vi "Set Current.vi"(4 "Factor (50.00) (EIN)":dbl=50.0, 6 "A Sensor Ratio(mV/A) (10.0000)":dbl=10.0 min=0.0001 max=99999.9999 step=0.0001 format="%.4f", 8 "error in (no error)":errorcluster, 9 "A Range (9: 5A)":u16(ring)=9 items=["AUTO", "10 mA", "20 mA", "50 mA", "100 mA", "200 mA", "500 mA", "1 A", "2 A", "5 A", "10 A", "20 A", "50 A", "S-AUTO", "50 mV", "100 mV", "250 mV", "500 mV", "1 V", "2.5 V", "5 V", "10 V"], 10 "Element (0: All)":u16(ring) items=["All", "Element 1", "Element 2", "Element 3", "Element 4", "Element 5", "Element 6"], 11 "Universal Power Meter in":refnum<class "Universal Power Meter.lvclass">) -> (0 "error out":errorcluster, 2 "Power Meter Visa":refnum<visa-resource-name>, 3 "Universal Power Meter out":refnum<class "Universal Power Meter.lvclass">)   [LabVIEW 2014, in "Universal Power Meter.lvlib" / "Universal Power Meter.lvclass"]
uses:
  Universal Power Meter.lvclass
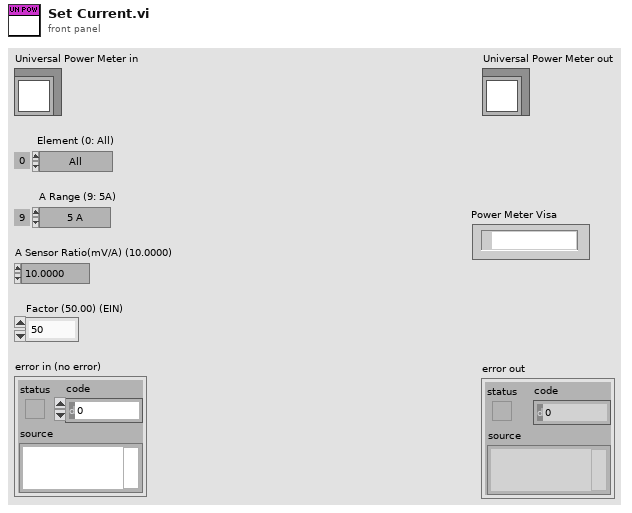
[diagram p1: front panel]
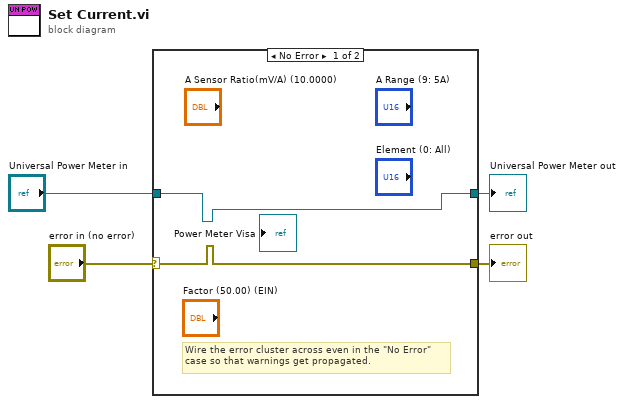
[diagram p0: block diagram]
diagram:
  n1 = case shown="No Error" "error in (no error)" {
    selector: "error in (no error)" -> [w5 w8]
    tunnel: [w5 w8] -> w3
    tunnel: [w6 w7] -> w1
    tunnel: "Universal Power Meter in" -> [w6 w7]
    frame No Error {
      # "Wire the error cluster across even in the \"No Error\"\ncase so that warnings get propagated."
    }
    frame Error {
    }
  }
  "error out" <- w3
  "Universal Power Meter out" <- w1
